vi "constructor.vi"(10 "Beverage.lvclass":refnum<class "Beverage.lvclass">, 11 "Soy in":refnum<class "Soy.lvclass">) -> (3 "Soy out":refnum<class "Soy.lvclass">)   [LabVIEW 2020, in "Soy.lvclass"]
uses:
  Soy.lvclass
  Beverage.lvclass
  Soy.lvclass/Soy.ctl
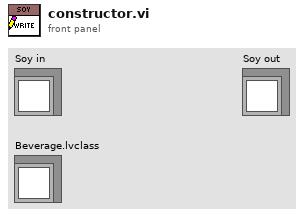
[diagram p1: front panel]
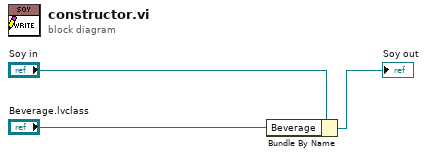
[diagram p0: block diagram]
diagram:
  n1 = Bundle By Name(cluster="Soy in", "Beverage"="Beverage.lvclass") -> (→"Soy out":refnum<class "Soy.lvclass">)
